vi "QueueUnderstanding.vi"() -> ()   [LabVIEW 2017]
uses:
  Subsystem/Subsystem.lvclass
panel:
  out "Over Max Timeout?":bool
  out "last update time":timestamp
  in  "stop 2":bool
  out "current time 2":timestamp
  out "current time":timestamp
  in  "stop":bool
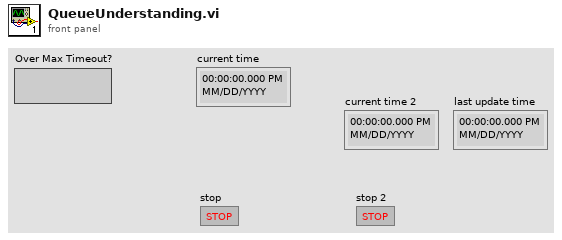
[diagram p1: front panel]
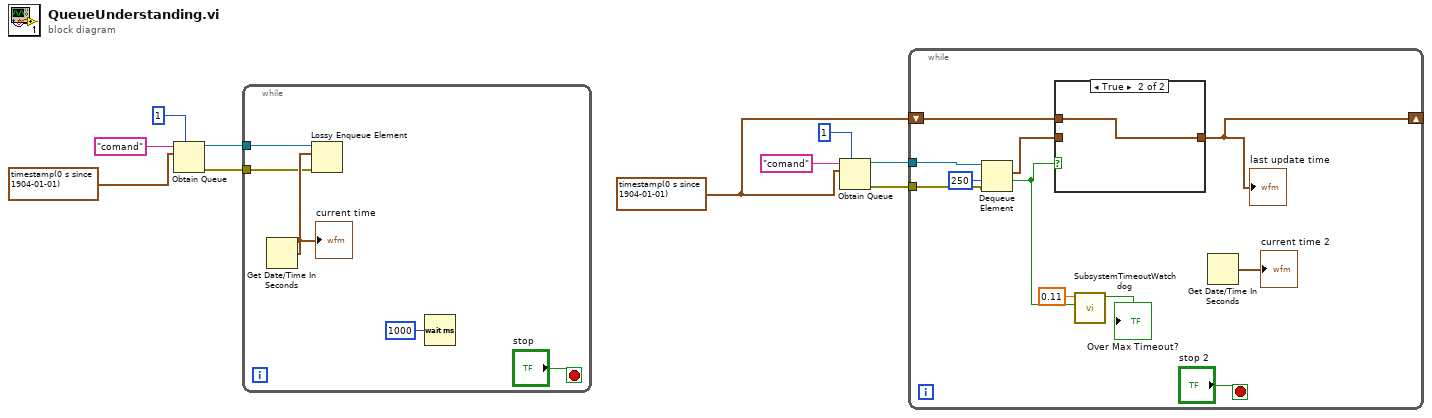
[diagram p0: block diagram]
diagram:
  w1 = timestamp(0 s since 1904-01-01)
  n1 = Obtain Queue(max queue size (-1, unlimited)=1, name (unnamed)="comand", element data type=timestamp(0 s since 1904-01-01)) -> (queue out=w7:refnum<queue>, error out=w6:errorcluster)  [unwired: 2 in, 1 out]
  n2 = while {
    tunnel: w7 -> [w13]
    tunnel: w6 -> [w12]
    stop <- "stop" stop-if-true
    n3 = Get Date/Time In Seconds() -> (seconds since 1Jan1904=w14:timestamp)
    "current time" <- w14
    n4 = Lossy Enqueue Element(queue=w13, element=w14, error in (no error)=w12) -> ()  [unwired: 4 out]
    n5 = Wait (ms)(milliseconds to wait=u32 1000) -> ()  [unwired: 1 out]
  }
  n6 = Obtain Queue(max queue size (-1, unlimited)=1, name (unnamed)="comand", element data type=w1) -> (queue out=w3:refnum<queue>, error out=w2:errorcluster)  [unwired: 2 in, 1 out]
  n7 = while {
    tunnel: w3 -> [w25]
    tunnel: w2 -> [w24]
    shift-right: [w19] -> _
    shift-left: w1 -> [w21]
    stop <- "stop 2" stop-if-true
    n8 = Dequeue Element(queue=w25, timeout in ms (-1)=250, error in (no error)=w24) -> (element=w22:timestamp, timed out?=w17:bool)  [unwired: 2 out]
    n9 = case shown="True" w17 {
      tunnel: [w27 w28] -> w19
      tunnel: w22 -> [w27 _]
      tunnel: w21 -> [_ w28]
      frame False {
      }
      frame True {
      }
    }
    "last update time" <- w19
    n10 = call "SubsystemTimeoutWatchdog.vi"("Keep counting?"=w17, "Max Timeout (s)"=0.11) -> ("Over Max Timeout?"=→"Over Max Timeout?":bool)  [unwired: 9 in]
    n11 = Get Date/Time In Seconds() -> (seconds since 1Jan1904=→"current time 2":timestamp)
  }
